vi "Generate Template Waveform.vi"(0 "signal configuration":refnum<class "SV Signal.lvclass">, 1 "reset":bool, 9 "number of samples":i32, 11 "error in (no error)":errorcluster) -> (4 "signal configuration":refnum<class "SV Signal.lvclass">, 6 "output waveform":waveform(dbl), 10 "samples this segment":i32, 15 "error out":errorcluster)   [LabVIEW 2017, in "SV Signal.lvclass"]
uses:
  <vilib>/addons/_NISVFA/_Generation/Signal Generation/SV Signal/SV Signal.lvclass
  <vilib>/addons/_NISVFA/_Generation/Signal Generation/SV Signal/sv_Generation State.ctl
  <vilib>/addons/_NISVFA/_Generation/Signal Generation/SV Signal/SV Signal.lvclass/SV Signal.ctl
  <vilib>/addons/_NISVFA/_Generation/Signal Generation/SV Function/SV Function.lvclass
panel:
  out "generation state":T1
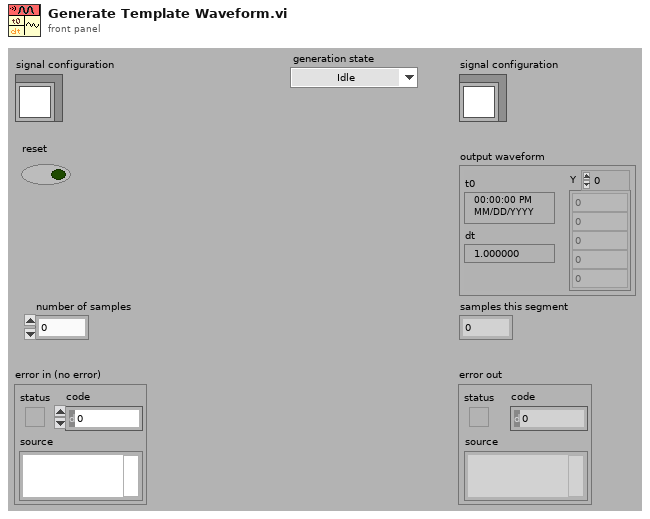
[diagram p1: front panel]
types:
  T1 = typedef "SV Signal.lvclass/sv_Generation State.ctl" = enum16{"Idle", "Ramp Up", "Pre-Measurement Settling", "Measurement", "Post-Measurement Settling", "Discrete Sweep Transition", "Ramp Down", "Update"}
  T2 = typedef "SV Signal.lvclass/sv_System Timing Model.ctl" = i64
  T3 = cluster{"system timing model":T2, "state":cluster{"RESET":bool, "generator timestamp":timestamp, "elapsed seconds":dbl, "elapsed samples":u64, "generation state":T1, "time offset at state":dbl, "samples generated at state":u64, "signal state":variant}, "duration of state":dbl, "samples remaining at state":i32}
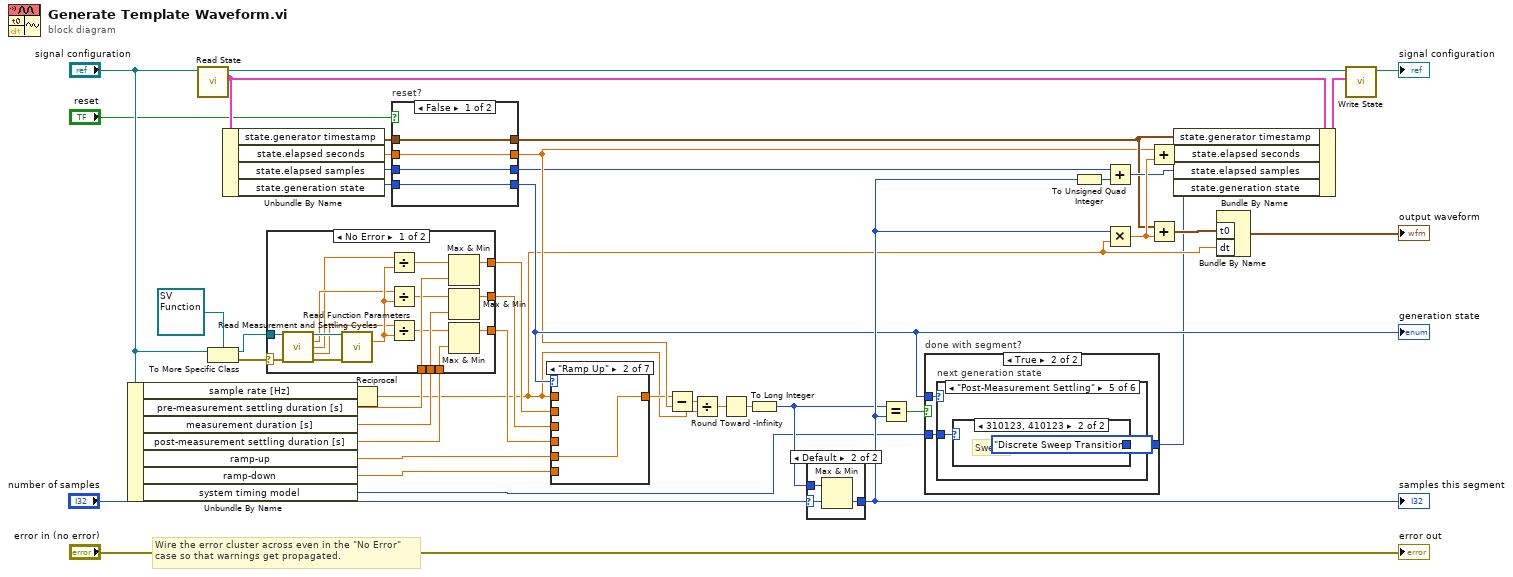
[diagram p0: block diagram]
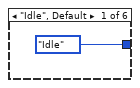
[diagram p3: hidden frame]
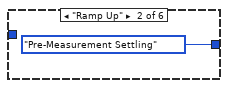
[diagram p4: hidden frame]
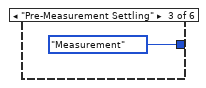
[diagram p5: hidden frame]
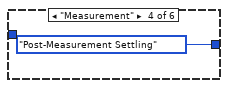
[diagram p6: hidden frame]
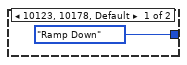
[diagram p7: hidden frame]
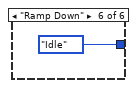
[diagram p8: hidden frame]
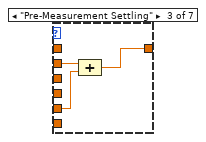
[diagram p11: hidden frame]
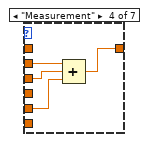
[diagram p12: hidden frame]
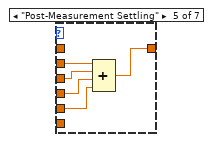
[diagram p13: hidden frame]
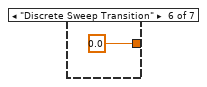
[diagram p14: hidden frame]
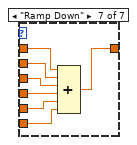
[diagram p15: hidden frame]
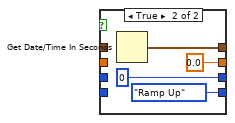
[diagram p17: hidden frame]
diagram:
  # "Wire the error cluster across even in the \"No Error\"\ncase so that warnings get propagated."
  n1 = Unbundle By Name("signal configuration") -> ("sample rate [Hz]"=w36:dbl, "pre-measurement settling duration [s]"=w22:dbl, "measurement duration [s]"=w23:dbl, "post-measurement settling duration [s]"=w21:dbl, "ramp-up"=w12:dbl, "ramp-down"=w25:dbl, "system timing model"=w3:T2)
  n2 = call <vilib>:"Read State.vi"("signal configuration"="signal configuration") -> ("generator state"=w28:T3, "signal configuration"=w34:refnum<class "SV Signal.lvclass">)  [unwired: 8 in, 1 out]
  n3 = To More Specific Class(target class=refnum<class "SV Function.lvclass"> refnum ("SV Function.lvclass"), reference="signal configuration") -> (specific class reference=w16:refnum<class "SV Function.lvclass">, error out=w17:errorcluster)  [unwired: 1 in]
  n4 = Unbundle By Name(w28) -> ("state.generator timestamp"=w35:timestamp, "state.elapsed seconds"=w31:dbl, "state.elapsed samples"=w30:u64, "state.generation state"=w15:T1)
  n5 = case shown="No Error" w17 {
    selector: w17 -> [w46 _]
    tunnel: w23 -> [w56 w63]
    tunnel: w22 -> [w55 w64]
    tunnel: w21 -> [w54 w62]
    tunnel: [w53 w62] -> w20
    tunnel: [w52 w63] -> w19
    tunnel: [w51 w64] -> w18
    tunnel: w16 -> [w47 _]
    frame No Error {
      n6 = call <vilib>:"Read Measurement and Settling Cycles.vi"("signal configuration"=w47, "error in (no error)"=w46) -> ("signal configuration"=w61:refnum<class "SV Function.lvclass">, "measurement cycles"=w59:dbl, "pre-measurement settling cycles"=w58:dbl, "post-measurement settling cycles"=w57:dbl, "error out"=w45:errorcluster)  [unwired: 9 in]
      n7 = call <vilib>:"Read Function Parameters.vi"("signal configuration"=w61, "error in (no error)"=w45) -> ("frequency_Hz"=w60:dbl)  [unwired: 8 in, 5 out]
      n8 = Divide(x=w58, y=w60) -> (x/y=w49:dbl)
      n9 = Divide(x=w59, y=w60) -> (x/y=w50:dbl)
      n10 = Divide(x=w57, y=w60) -> (x/y=w48:dbl)
      n11 = Max & Min(x=w49, y=w55) -> (max(x,y)=w51:dbl)  [unwired: 1 out]
      n12 = Max & Min(x=w50, y=w56) -> (max(x,y)=w52:dbl)  [unwired: 1 out]
      n13 = Max & Min(x=w48, y=w54) -> (max(x,y)=w53:dbl)  [unwired: 1 out]
    }
    frame Error {
    }
  }
  n14 = Reciprocal(x=w36) -> (1/x=w7:dbl)
  n15 = case "reset?" shown="False" "reset" {
    tunnel: w35 -> [w68 _]
    tunnel: [w68 w72] -> w26
    tunnel: [w67 0.0 ("TimeSinceLastReset")] -> w14
    tunnel: [w66 u64 0 ("elapsed samples")] -> w13
    tunnel: w31 -> [w67 _]
    tunnel: w30 -> [w66 _]
    tunnel: w15 -> [w65 _]
    tunnel: [w65 sv_Generation_State."Ramp Up" ("generation state")] -> w38
    frame False {
    }
    frame True {
      n16 = Get Date/Time In Seconds() -> (seconds since 1Jan1904=w72:timestamp)
    }
  }
  "generation state" <- w38
  n17 = case shown="\"Ramp Up\"" w38 {
    tunnel: w7 -> [w73 _ _ _ _ _ w90]
    tunnel: w12 -> [_ w74 w77 w78 w82 _ w88]
    tunnel: w18 -> [_ _ w76 w81 w86 _ w94]
    tunnel: w19 -> [_ _ _ w80 w85 _ w93]
    tunnel: w20 -> [_ _ _ _ w84 _ w92]
    tunnel: w25 -> [_ _ _ _ _ _ w91]
    tunnel: [w73 w74 w75 w79 w83 0.0 ("ramp down time [s]") w89] -> w11
    frame "Idle", Default {
    }
    frame "Ramp Up" {
    }
    frame "Pre-Measurement Settling" {
      n18 = Compound Arithmetic op=ADD(w76, w77) -> (w75:dbl)
    }
    frame "Measurement" {
      n19 = Compound Arithmetic op=ADD(w81, w80, w78) -> (w79:dbl)
    }
    frame "Post-Measurement Settling" {
      n20 = Compound Arithmetic op=ADD(w86, w85, w84, w82) -> (w83:dbl)
    }
    frame "Discrete Sweep Transition" {
    }
    frame "Ramp Down" {
      n21 = Compound Arithmetic op=ADD(w90, w94, w93, w92, w88, w91) -> (w89:dbl)
    }
  }
  n22 = Subtract(x=w11, y=w14) -> (x-y=w10:dbl)
  n23 = Divide(x=w10, y=w7) -> (x/y=w9:dbl)
  n24 = Round Toward -Infinity(1:w9) -> (0:w8:dbl)
  n25 = To Long Integer(number=w8) -> (32bit integer=w5:i32)
  n26 = case shown="Default" "number of samples" {
    selector: "number of samples" -> [_ w97]
    tunnel: w5 -> [w95 w98]
    tunnel: [w95 w96] -> w40
    frame ..-1 {
    }
    frame Default {
      n27 = Max & Min(x=w98, y=w97) -> (min(x,y)=w96:i32)  [unwired: 1 out]
    }
  }
  "samples this segment" <- w40
  n28 = Equal?(x=w5, y=w40) -> (x = y?=w4:bool)
  n29 = case "done with segment?" shown="True" w4 {
    tunnel: [w99 w102] -> w6
    tunnel: w3 -> [_ w101]
    tunnel: w38 -> [w99 w100]
    frame False {
    }
    frame True {
      n30 = case "next generation state" shown="\"Post-Measurement Settling\"" w100 {
        tunnel: w101 -> [_ _ _ _ w108 _]
        tunnel: [sv_Generation_State."Idle" ("generation state") sv_Generation_State."Pre-Measurement Settling" ("generation state") sv_Generation_State."Measurement" ("generation state") sv_Generation_State."Post-Measurement Settling" ("generation state") w107 sv_Generation_State."Idle" ("generation state")] -> w102
        frame "Idle", Default {
        }
        frame "Ramp Up" {
        }
        frame "Pre-Measurement Settling" {
        }
        frame "Measurement" {
        }
        frame "Post-Measurement Settling" {
          n31 = case shown="310123, 410123" w108 {
            tunnel: [sv_Generation_State."Ramp Down" ("generation state") sv_Generation_State."Discrete Sweep Transition" ("generation state")] -> w107
            frame 10123, 10178, Default {
            }
            frame 310123, 410123 {
              # "Sweep"
            }
          }
        }
        frame "Ramp Down" {
        }
      }
    }
  }
  n32 = To Unsigned Quad Integer(1:w40) -> (0:w27:u64)
  n33 = Add(x=w13, y=w27) -> (x+y=w32:u64)
  n34 = Multiply(x=w40, y=w7) -> (x*y=w37:dbl)
  n35 = Add(x=w14, y=w37) -> (x+y=w33:dbl)
  n36 = Add(x=w26, y=w37) -> (x+y=w29:timestamp)
  n37 = Bundle By Name(cluster=w28, "state.generator timestamp"=w26, "state.elapsed seconds"=w33, "state.elapsed samples"=w32, "state.generation state"=w6) -> (w2:T3)
  n38 = Bundle By Name("t0"=w29, "dt"=w7) -> (→"output waveform":waveform(dbl))  [unwired: 1 in]
  n39 = call <vilib>:"Write State.vi"("generator state"=w2, "signal configuration"=w34) -> ("signal configuration"=→"signal configuration":refnum<class "SV Signal.lvclass">)  [unwired: 8 in, 1 out]
  "error out" <- "error in (no error)"
